vi "CLD3 FGV Timer no pause front panel.vi"(8 "Fehler (Eingang, kein Fehler)":errorcluster, 10 "Warten":dbl, 11 "Timer-Task":T1) -> (0 "Fehler (Ausgang)":errorcluster, 2 "Verstrichene Zeit?":bool, 3 "Verstrichene Zeit":dbl)   [LabVIEW 2009]
doc: "CLD-Zusatzaufgabe 3"
uses:
  CLD3 Timer Mode.ctl
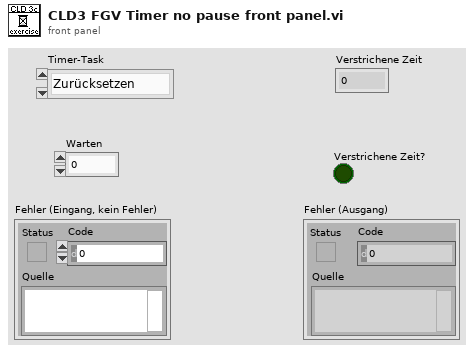
[diagram p1: front panel]
types:
  T1 = typedef "CLD3 Timer Mode.ctl" = enum16{"Zurücksetzen", "Verstrichen"}
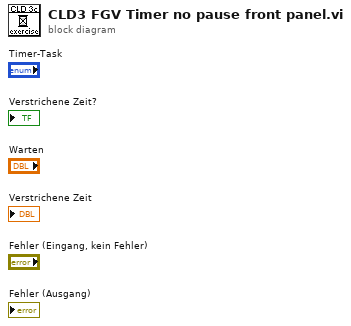
[diagram p0: block diagram]
diagram:
